vi "ClearParameter.vi"(1 "Parameter":string) -> (0 "Error":bool)   [LabVIEW 2014]
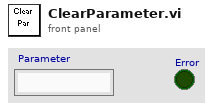
[diagram p1: front panel]
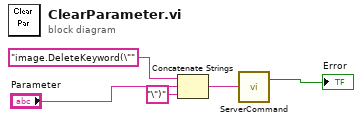
[diagram p0: block diagram]
diagram:
  n1 = Concatenate Strings("image.DeleteKeyword(\"" ("Command"), "Parameter", "\")" ("string")) -> (w2:string)
  n2 = call "ServerCommand.vi"("Command"=w2) -> ("Error"=→"Error":bool)  [unwired: 1 out]
